vi "Charger_Is State Match.vi"(1 "ChargeRecord":T1={"ChargingState"="CHARGE_PRE_CONDITION-1", "Temp"=enum."LE 3", "Low Limit"=-inf, "High Limit"=225.0, "Charger"=enum."Adjust", "Adjustment"=-100.0} {"High Limit" format="%.1f"; "Low Limit" format="%.1f"; "Adjustment" format="%.1f"}, 2 "ReceivedLevel":dbl format="%.1f", 3 "TemperatureLevel":dbl, 4 "ChargingState":string="CHARGE_OFF-0") -> (0 "Match":bool)   [LabVIEW 2020]
doc: "This function compares a Charging State, Temperature Level, and Received Level to a \"Charger Next Action\" cluster to determine the match status."
uses:
  Charger_Next_Action.ctl
  Charger_States_Control.ctl
panel:
  # "ChargingState"
  # "Temp"
  # "Low Limit"
  # "High Limit"
  # "Charger"
  # "Adjustment"
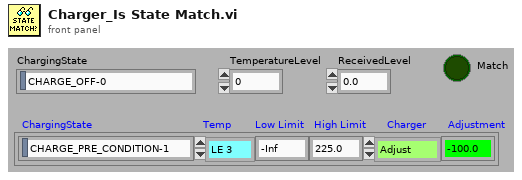
[diagram p1: front panel]
types:
  T1 = typedef "Charger_Next_Action.ctl" = cluster{"ChargingState":string, "Temp":enum16{"Any", "GT 3", "LE 3", "GT 2", "LE 2"}, "Low Limit":dbl, "High Limit":dbl, "Charger":T2, "Adjustment":dbl}
  T2 = typedef "Charger_States_Control.ctl" = enum16{"Enable", "Disable", "Adjust", "Pause", "na"}
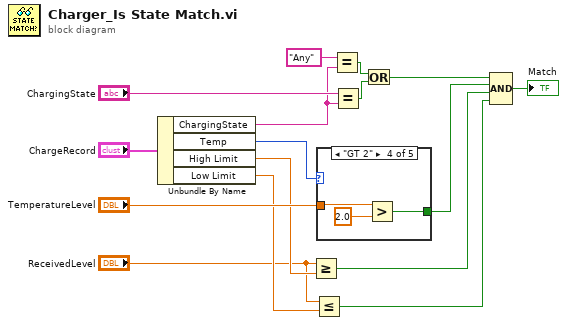
[diagram p0: block diagram]
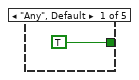
[diagram p2: hidden frame]
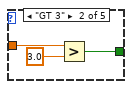
[diagram p3: hidden frame]
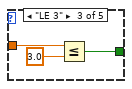
[diagram p4: hidden frame]
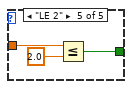
[diagram p5: hidden frame]
diagram:
  n1 = Unbundle By Name("ChargeRecord") -> ("ChargingState"=w1:string, "Temp"=w7:enum16{"Any", "GT 3", "LE 3", "GT 2", "LE 2"}, "High Limit"=w6:dbl, "Low Limit"=w5:dbl)
  n2 = Greater Or Equal?(x="ReceivedLevel", y=w6) -> (x >= y?=w3:bool)
  n3 = Less Or Equal?(x="ReceivedLevel", y=w5) -> (x <= y?=w2:bool)
  n4 = case shown="\"GT 2\"" w7 {
    tunnel: "TemperatureLevel" -> [_ w18 w23 w26 w29]
    tunnel: [TRUE w20 w21 w24 w27] -> w8
    frame "Any", Default {
    }
    frame "GT 3" {
      n5 = Greater?(x=w18, y=3.0) -> (0:w20:bool)
    }
    frame "LE 3" {
      n6 = Less Or Equal?(x=w23, y=3.0) -> (x <= y?=w21:bool)
    }
    frame "GT 2" {
      n7 = Greater?(x=w26, y=2.0) -> (0:w24:bool)
    }
    frame "LE 2" {
      n8 = Less Or Equal?(x=w29, y=2.0) -> (x <= y?=w27:bool)
    }
  }
  n9 = Equal?(x="Any", y=w1) -> (x = y?=w13:bool)
  n10 = Equal?(x="ChargingState", y=w1) -> (x = y?=w14:bool)
  n11 = Or(x=w13, y=w14) -> (x .or. y?=w9:bool)
  n12 = Compound Arithmetic op=AND(w9, w8, w3, w2) -> (→"Match":bool)
